vi "MAIN_merFSIH_scan_brightfield.vi"(5 "queue CAMERA":refnum<queue>, 7 "queue piezo":refnum<queue>, 8 "error in":errorcluster, 9 "Display?":bool=TRUE, 10 "Exp time (s)":sgl=0.05 format="%#_3g", 11 "DATA cluster":T1) -> (0 "error out":errorcluster, 3 "Next task":T2)   [LabVIEW 2015]
uses:
  CONTROLS/Q_MCL_piezo_element.ctl
  GLOBAL/Global_ABORT.vi
  GLOBAL/Global_MAIN.vi
  GLOBAL/Global_MCL_piezo.vi
  CONTROLS/Q_camera_element.ctl
  CONTROLS/Q_main_element.ctl
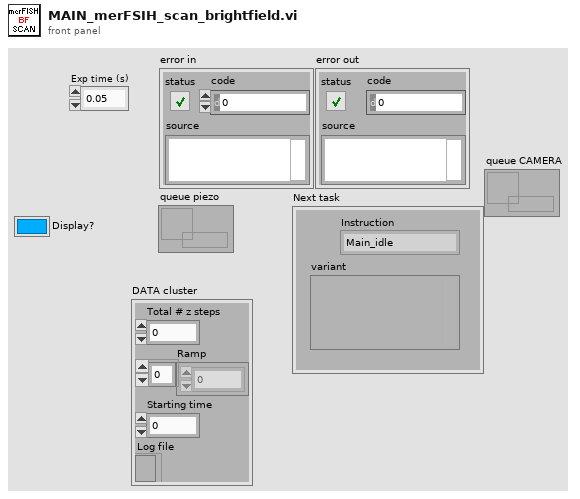
[diagram p1: front panel]
types:
  T1 = cluster{"Total # z steps":i32, "Ramp":dbl[], "Starting time":dbl, "Log file":refnum<file>}
  T2 = typedef "Q_main_element.ctl" = cluster{"variant":variant, "Instruction":enum16{"Main_idle", "Main_initialize", "Main_initialize_TDMS", "Main_initialize_Queue", "Main_error", "Main_DAQ_initialization_results", "Main_ASI_initialization_results", "Main_Piezo_initialization_results", "Main_Valve_initialization_results", "Main_Pump_initialization_results", "Main_CAMERA_initialization_results", "Main_FPGA_initialization_results", "Main_DAQ_error", "Main_ASI_error", "Main_Piezo_error", "Main_CAMERA_error", "Main_Valve_error", "Main_Pump_error", "Main_FPGA_error", "Main_start_acquiring", "Main_not_acquiring", "Main_acquiring", "Main_stop_acquiring", "Main_change_exposure", "Main_change_z_scan_parameters", "Main_define_ROI", "Main_define_mosaic", "Main_read_kinetic_time", "Main_cooler", "Main_read_temperature", "Main_save_XY", "Main_load_XY", "Main_discard_XY", "Main_move_to_XY", "Main_measure_QPD", "Main_autofocus_calibration", "Main_autofocus_initialization", "Main_autofocus_stop", "Main_save_PID", "Main_change_H_valve_position", "Main_two_way_valve", "Main_save_movie", "Main_init_single_scan", "Main_single_scan", "Main_stop_single_scan", "Main_merFISH_illumination_parameters", "Main_merFISH_buffer_probe_list", "Main_merFISH_injections_procedure", "Main_merFISH_save_setpoint", "Main_merFISH_DAPI_parameters", "Main_merFISH_Brightfield_parameters", "Main_merFISH_save_embryo_ROI", "Main_merFISH_init", "Main_merFISH_resume", "Main_merFISH_start_autofocus", "Main_merFISH_open_close_valve_merFISH", "Main_merFISH_open_close_valve_photobleaching", "Main_merFISH_hybridization", "Main_merFISH_move_to_ROI", "Main_merFISH_wait_stabilization", "Main_merFISH_scan_laser", "Main_merFISH_scan_brightfield", "Main_merFISH_photobleaching_injection", "Main_merFISH_photobleaching", "Main_merFISH_save", "Main_merFISH_send_email", "Main_merFISH_close", "Main_STOP"}}
  T3 = typedef "Q_MCL_piezo_element.ctl" = cluster{"variant":variant, "Instruction":enum16{"Piezo_idle", "Piezo_initialize", "Piezo_error", "Piezo_security_stop", "Piezo_read_z", "Piezo_move_z", "Piezo_keyboard_move", "Piezo_close_autofocus_calibration_ramp", "Piezo_change_init_state", "Piezo_init_autofocus", "Piezo_init_autofocus_merFISH_TL", "Piezo_autofocus", "Piezo_autofocus_merFISH_TL", "Piezo_stop_autofocus", "Piezo_stop_autofocus_merFISH_TL", "Piezo_autofocus_lost", "Piezo_resume_autofocus_merFISH_TL", "Piezo_check_z_position_merFISH_TL", "Piezo_init_ramp", "Piezo_move_z_ramp", "Piezo_close_ramp", "Piezo_close_merFISH", "Piezo_stop"}}
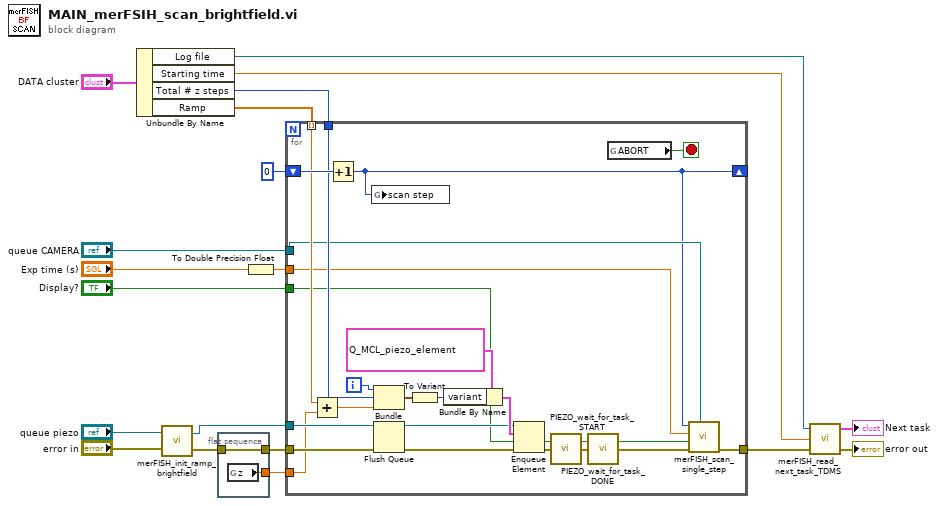
[diagram p0: block diagram]
diagram:
  n1 = Unbundle By Name("DATA cluster") -> ("Log file"=w3:refnum<file>, "Starting time"=w4:dbl, "Total # z steps"=w17:i32, "Ramp"=w18:dbl[])
  n2 = call "merFISH_init_ramp_brightfield.vi"("error in"="error in", "Piezo queue"="queue piezo") -> ("error out"=w8:errorcluster, "Piezo queue out"=w5:refnum<queue>)
  n3 = flat-sequence {
    tunnel: [w21] -> w10
    tunnel: w8 -> [w20]
    tunnel: [w20] -> w11
    frame #0 {
      n4 = global read "Global_MCL_piezo.vi" "z"() -> (w21:dbl)
    }
  }
  n5 = To Double Precision Float(number="Exp time (s)") -> (double precision float=w9:dbl)
  n6 = for {
    tunnel: w18 -> [w27] mode=indexing
    tunnel: w17 -> [w35]
    shift-right: [w22] -> _
    shift-left: 0 -> [w37]
    tunnel: [w34] -> w2
    tunnel: w5 -> [w32]
    tunnel: w11 -> [w31]
    tunnel: w9 -> [w26]
    tunnel: w10 -> [w25]
    tunnel: "Display?" -> [w24]
    tunnel: "queue CAMERA" -> [w23]
    i -> [w38]
    stop <- w33 stop-if-true
    n7 = Add(x=w27, y=w25) -> (x+y=w28:dbl)
    n8 = Increment(x=w37) -> (x+1=w22:i32)
    n9 = global write "Global_MAIN.vi" "scan step"(w22) -> ()
    n10 = Bundle(w38, "Total # z steps"=w35, w28) -> (w44:cluster{i32, "Total # z steps":i32, dbl})  [unwired: 1 in]
    n11 = Flush Queue(queue=w32, error in (no error)=w31) -> (queue out=w30:refnum<queue>, error out=w29:errorcluster)  [unwired: 1 out]
    n12 = To Variant(anything=w44) -> (Variant=w40:variant)
    n13 = Bundle By Name(cluster=T3 {"variant"=variant, "Instruction"=enum."Piezo_move_z_ramp"} ("Q_MCL_Piezo"), "variant"=w40) -> (w41:T3)
    n14 = Enqueue Element(queue=w30, element=w41, error in (no error)=w29) -> (error out=w42:errorcluster)  [unwired: 1 in, 2 out]
    n15 = call "PIEZO_wait_for_task_START.vi"("error in"=w42) -> ("error out"=w43:errorcluster)
    n16 = call "PIEZO_wait_for_task_DONE.vi"("error in"=w43) -> ("error out"=w36:errorcluster)
    n17 = global read "Global_ABORT.vi" "ABORT"() -> (w33:bool)
    n18 = call "merFISH_scan_single_step.vi"("queue DAQ"=w23, "error in"=w36, "Z position"=w24, "# steps"=w26, "queue piezo"=w22) -> ("error out"=w34:errorcluster)  [unwired: 3 in]
  }
  n19 = call "merFISH_read_next_task_TDMS.vi"("error in"=w2, "Starting time"=w4, "Log file"=w3) -> ("error out"=→"error out":errorcluster, "task"=→"Next task":T2)  [unwired: 1 in]
